vi "Tree.vi"() -> ()   [LabVIEW 2019, in "xy_utilities.lvlib"]
uses:
  xy_utilities.lvlib
  <vilib>/Analysis/NI_AALPro.lvlib
  <vilib>/Analysis/NI_AALBase.lvlib
  <vilib>/measure/NI_MAPro.lvlib
  subVIs/Waveform to XY (single).vi
  subVIs/Waveform to XY (multiple).vi
  subVIs/Interpolate (multiple).vi
  <vilib>/Analysis/6fits.llb/Remove Outliers (Range).vi
  <vilib>/ptbypt/NI_PtbyPt.lvlib
  subVIs/Shift Zero (single).vi
  subVIs/Decimate (single).vi
  subVIs/Subtract float (single).vi
  subVIs/Divide XY (single).vi
  subVIs/Remove Outliers (multiple).vi
  subVIs/Symmetrize (single).vi
  <vilib>/Waveform/WDTOps.llb/WDT Append Waveforms DBL.vi
  <vilib>/Analysis/3filter.llb/Zero Phase Filter (DBL).vi
  <vilib>/Analysis/baseanly.llb/Mean (DBL).vi
  subVIs/Append (double scaler).vi
  subVIs/Interpolate (single).vi
  subVIs/FFT (multiple).vi
  subVIs/Shift Zero (multiple).vi
  subVIs/Add XY (single).vi
  subVIs/Add XY (multiple).vi
  subVIs/XY to Waveform (single).vi
  subVIs/Interpolate Y (multiple).vi
  subVIs/Multiply XY (single).vi
  subVIs/Multiply float (multiple).vi
  subVIs/Square (multiple).vi
  subVIs/Subtract float (multiple).vi
  subVIs/Subset (single).vi
  subVIs/Reverse (multiple).vi
  subVIs/Zero Phase Lowpass Filter (single).vi
  subVIs/Decimate (multiple).vi
  subVIs/Divide float (multiple).vi
  subVIs/Symmetrize (multiple).vi
  subVIs/Restrict X Range (multiple).vi
  subVIs/Resample (single).vi
  subVIs/PS (single).vi
  subVIs/Subtract XY (single).vi
  subVIs/Multiply float (single).vi
  <vilib>/measure/maspectr.llb/FFT Spectrum (Mag-Phase) for 1 Chan.vi
  subVIs/Multiply XY (multiple).vi
  subVIs/Append (double array).vi
  subVIs/Divide XY (multiple).vi
  <vilib>/measure/maspectr.llb/FFT Power Spectrum and PSD for 1 Chan.vi
  subVIs/Get X and Y (single).vi
  subVIs/Remove Outliers (single).vi
  subVIs/FFT (single).vi
  subVIs/Sort (single).vi
  subVIs/Append (multiple).vi
  subVIs/Reverse (single).vi
  subVIs/Divide float (single).vi
  subVIs/Add float (multiple).vi
  subVIs/Savitsky Golay Filter (single).vi
  <vilib>/Analysis/2dsp.llb/Decimate (single shot, DBL).vi
  subVIs/Subset (multiple).vi
  subVIs/XY to Waveform (multiple).vi
  subVIs/Interpolate Y (single).vi
  subVIs/Restrict X Range (single).vi
  subVIs/Derivative (single).vi
  subVIs/Subtract XY (multiple).vi
  subVIs/Square (single).vi
  subVIs/PS (multiple).vi
  subVIs/Swap X and Y (single).vi
  subVIs/Sort (multiple).vi
  <vilib>/measure/maresamp.llb/Resample Waveform (single shot).vi
  subVIs/Resample (multiple).vi
  subVIs/Add float (single).vi
  subVIs/Append (single).vi
  subVIs/Derivative (multiple).vi
  subVIs/Moving Average (single).vi
  <vilib>/Analysis/3filter.llb/Savitzky-Golay Filter (DBL).vi
  subVIs/Swap X and Y (multiple).vi
  subVIs/Get X and Y (multiple).vi
  subVIs/Zero Phase Lowpass Filter (multiple).vi
  subVIs/Moving Average (multiple).vi
  subVIs/Savitsky Golay Filter (multiple).vi
  subVIs/Linear Fit (multiple).vi
  subVIs/Difference Quotient (multiple).vi
  subVIs/Difference Quotient (single).vi
  subVIs/Linear Fit (single).vi
panel:
  out "Array of XY-data":cluster{"X-array":dbl[], "Y-array":dbl[]}[](array[cluster])
  out "XY-data":cluster{"X-array":dbl[], "Y-array":dbl[]}
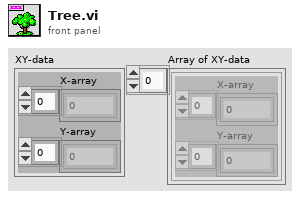
[diagram p1: front panel]
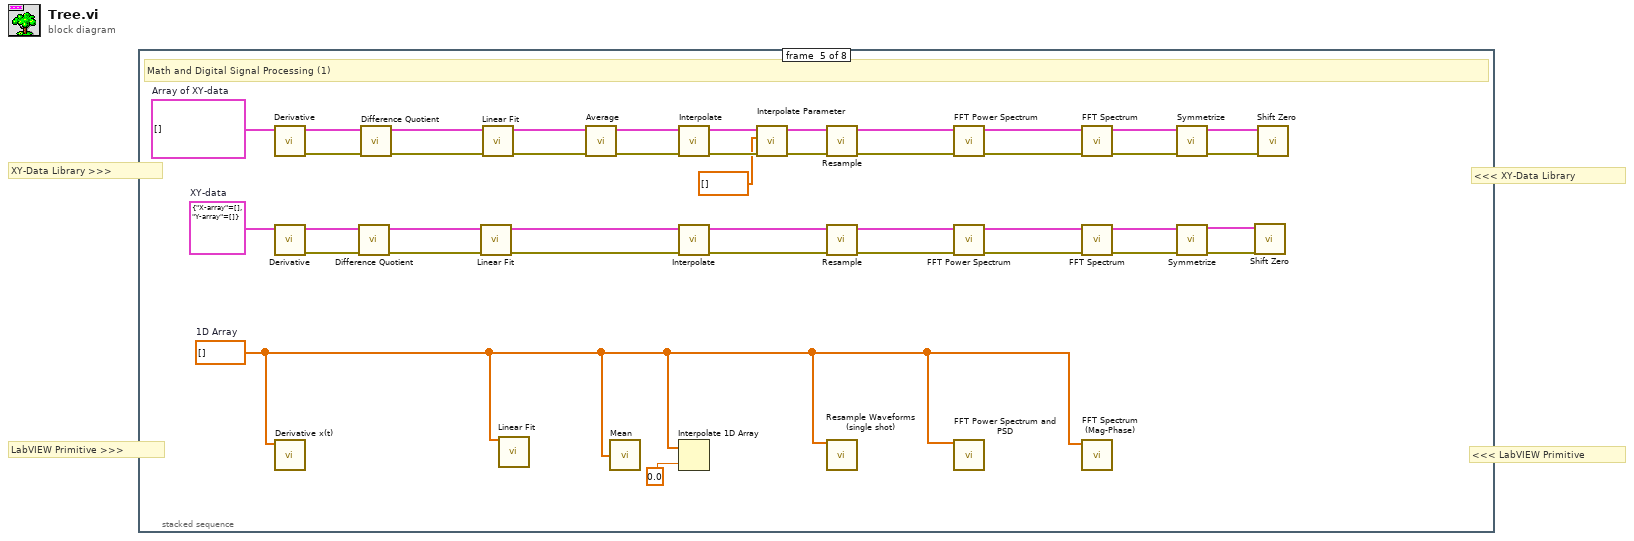
[diagram p0: block diagram]
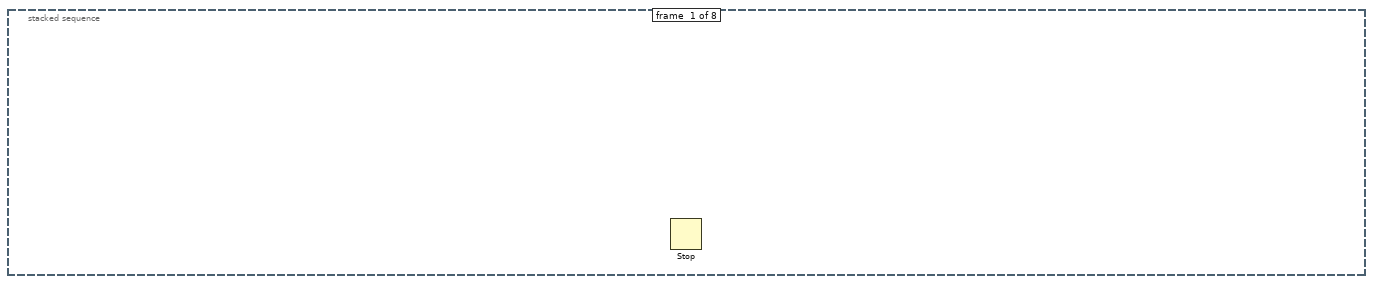
[diagram p2: hidden frame]
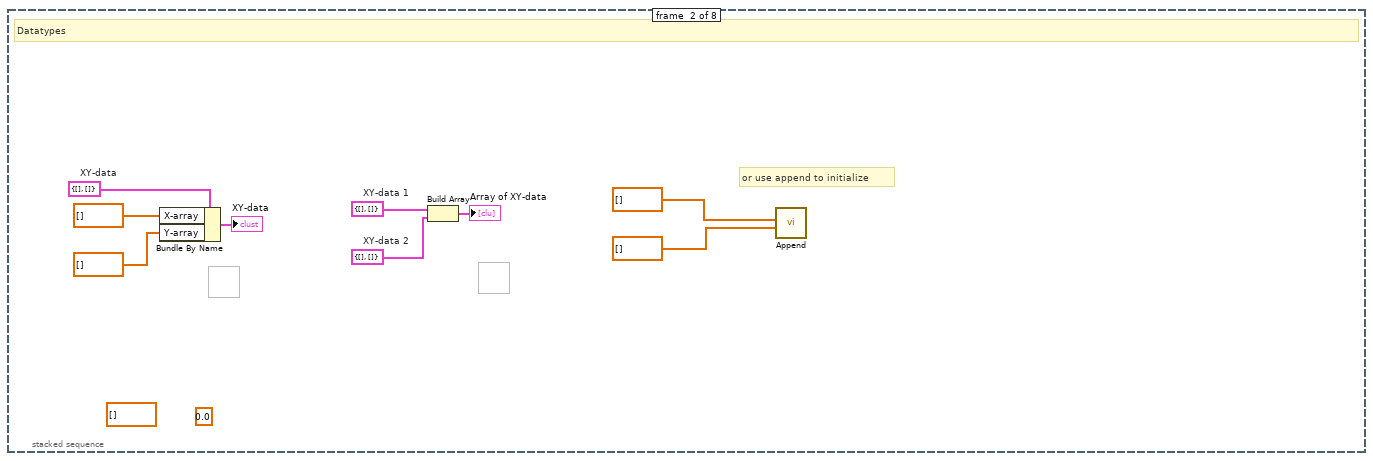
[diagram p3: hidden frame]
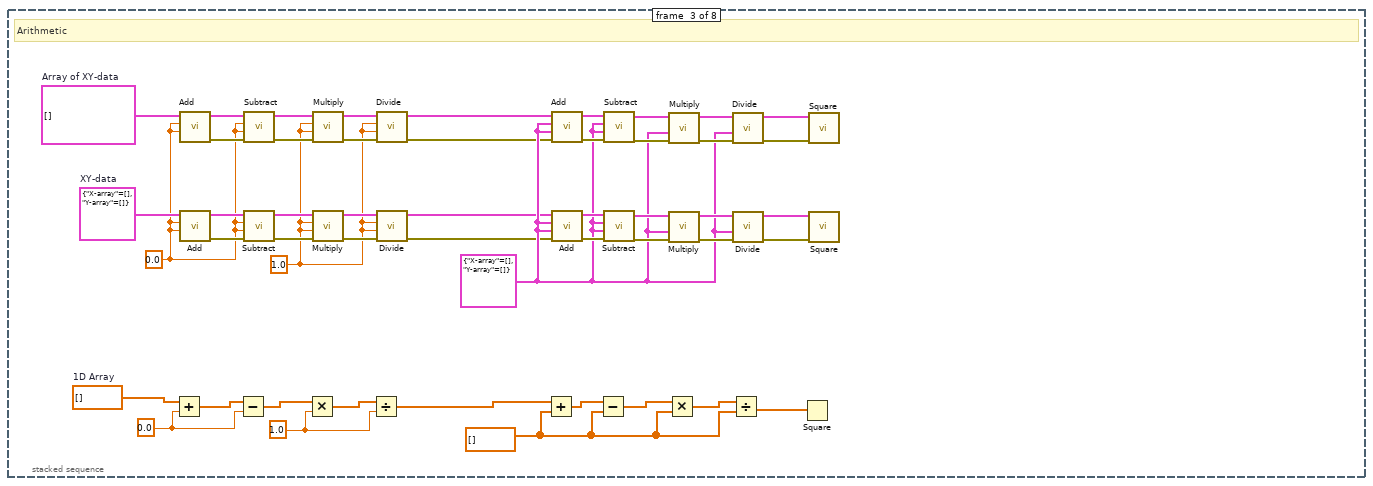
[diagram p4: hidden frame]
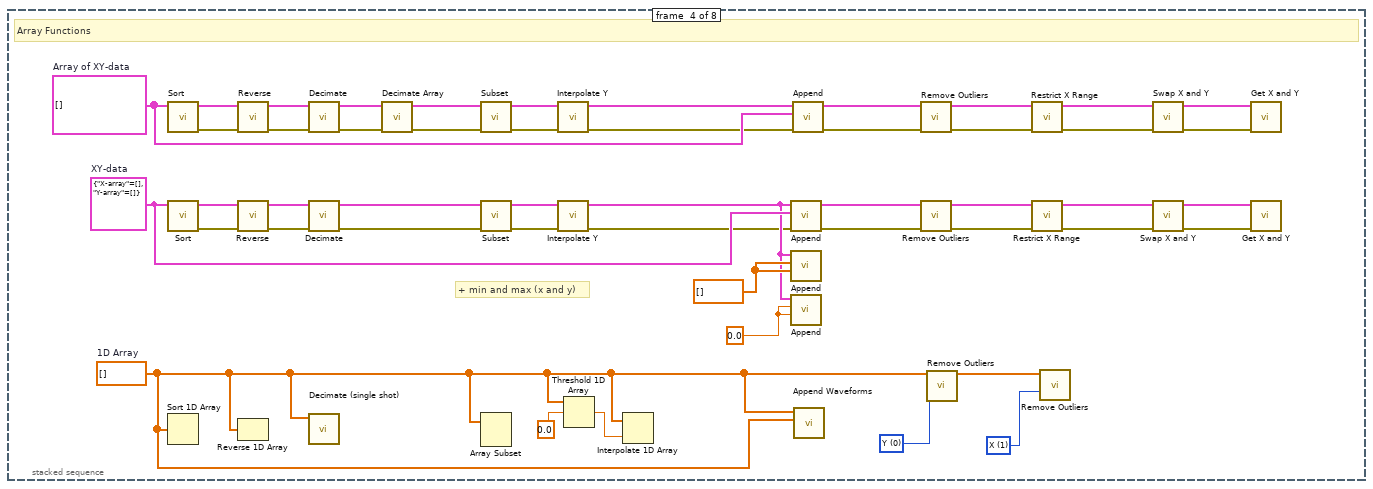
[diagram p5: hidden frame]
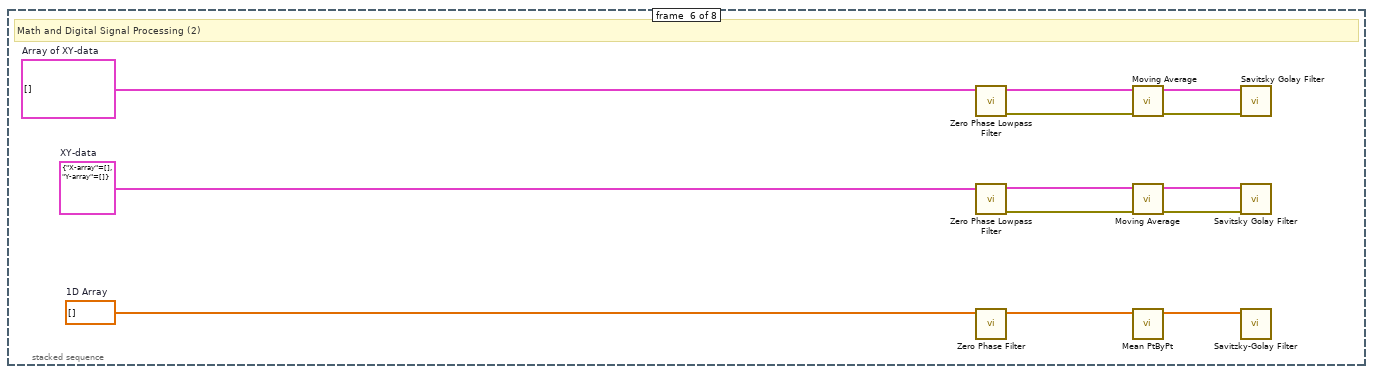
[diagram p6: hidden frame]
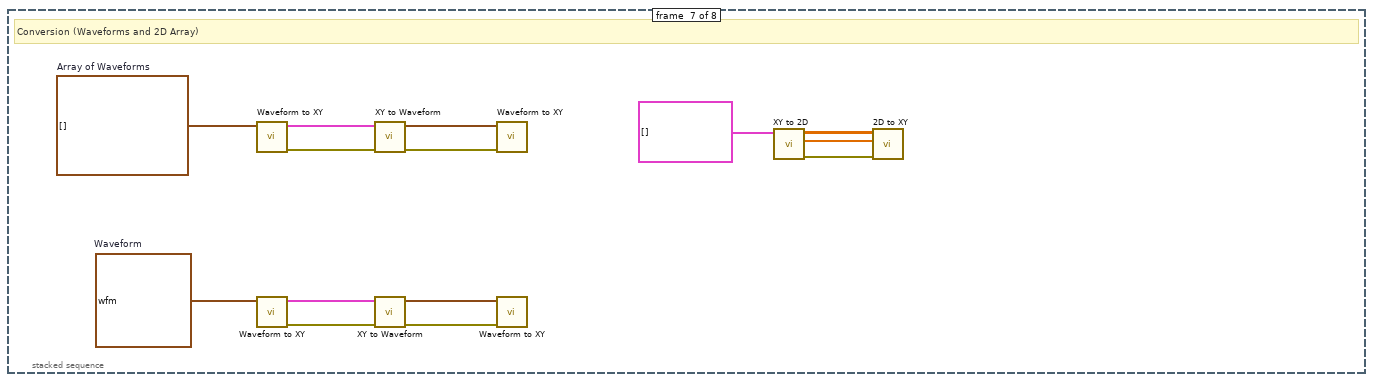
[diagram p7: hidden frame]
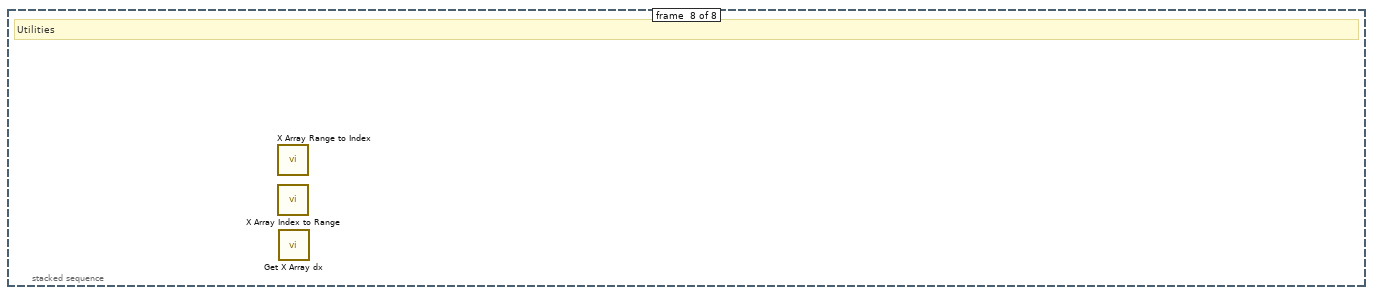
[diagram p8: hidden frame]
diagram:
  # "XY-Data Library >>>"
  # "LabVIEW Primitive >>>"
  # "<<< XY-Data Library"
  # "<<< LabVIEW Primitive"
  n1 = stacked-sequence {
    frame #0 {
      n2 = Stop() -> ()  [unwired: 1 in]
    }
    frame #1 {
      (unwired) 0.0
      (unwired) dbl[] [] ("Y-array")
      w7 = cluster{"X-array":dbl[], "Y-array":dbl[]} {"X-array"=[], "Y-array"=[]}  # XY-data 2
      w8 = cluster{"X-array":dbl[], "Y-array":dbl[]} {"X-array"=[], "Y-array"=[]}  # XY-data 1
      w6 = cluster{"X-array":dbl[], "Y-array":dbl[]} {"X-array"=[], "Y-array"=[]}  # XY-data
      # "or use append to initialize"
      # "Datatypes"
      n3 = Bundle By Name(cluster=w6, "X-array"=dbl[] [], "Y-array"=dbl[] []) -> (→"XY-data":cluster{"X-array":dbl[], "Y-array":dbl[]})
      n4 = Build Array(w8, w7) -> (→"Array of XY-data":cluster{"X-array":dbl[], "Y-array":dbl[]}[])
      n5 = call-poly "Append.vi"("Y-array"=dbl[] [], "X-array"=dbl[] []) -> ()  [unwired: 8 in, 2 out]
    }
    frame #2 {
      w24 = cluster{"X-array":dbl[], "Y-array":dbl[]} {"X-array"=[], "Y-array"=[]} ("XY-data in")
      w33 = 1.0 ("x (0)")
      w42 = 0.0 ("x (0)")
      w21 = dbl[] []
      w35 = 1.0 ("x (0)")
      w36 = 0.0 ("x (0)")
      w10 = dbl[] []  # 1D Array
      w58 = cluster{"X-array":dbl[], "Y-array":dbl[]}[] []  # Array of XY-data
      w57 = cluster{"X-array":dbl[], "Y-array":dbl[]} {"X-array"=[], "Y-array"=[]}  # XY-data
      # "Arithmetic"
      n6 = Add(x=w10, y=w36) -> (x+y=w56:dbl[])
      n7 = call-poly "Add.vi"("y (0)"=w42, "x (0)"=w42, "XY-data"=w58) -> ("error out"=w47:errorcluster, "XY-data out"=w48:cluster{"X-array":dbl[], "Y-array":dbl[]}[])  [unwired: 7 in]
      n8 = call-poly "Add.vi"("y (0)"=w42, "x (0)"=w42, "XY-data"=w57) -> ("error out"=w43:errorcluster, "XY-data out"=w44:cluster{"X-array":dbl[], "Y-array":dbl[]})  [unwired: 7 in]
      n9 = Subtract(x=w56, y=w36) -> (x-y=w55:dbl[])
      n10 = call-poly "Subtract.vi"("error in (no error)"=w47, "y (0)"=w42, "x (0)"=w42, "XY-data"=w48) -> ("error out"=w45:errorcluster, "XY-data out"=w46:cluster{"X-array":dbl[], "Y-array":dbl[]}[])  [unwired: 6 in]
      n11 = call-poly "Subtract.vi"("error in (no error)"=w43, "y (0)"=w42, "x (0)"=w42, "XY-data"=w44) -> ("error out"=w50:errorcluster, "XY-data out"=w51:cluster{"X-array":dbl[], "Y-array":dbl[]})  [unwired: 6 in]
      n12 = Multiply(x=w55, y=w35) -> (x*y=w37:dbl[])
      n13 = call-poly "Multiply.vi"("error in (no error)"=w45, "y (1)"=w33, "x (1)"=w33, "XY-data"=w46) -> ("error out"=w52:errorcluster, "XY-data out"=w54:cluster{"X-array":dbl[], "Y-array":dbl[]}[])  [unwired: 6 in]
      n14 = call-poly "Multiply.vi"("error in (no error)"=w50, "y (1)"=w33, "x (1)"=w33, "XY-data"=w51) -> ("error out"=w49:errorcluster, "XY-data out"=w53:cluster{"X-array":dbl[], "Y-array":dbl[]})  [unwired: 6 in]
      n15 = Divide(x=w37, y=w35) -> (x/y=w16:dbl[])
      n16 = call-poly "Divide.vi"("error in (no error)"=w52, "y (1)"=w33, "x (1)"=w33, "XY-data"=w54) -> ("error out"=w19:errorcluster, "XY-data out"=w20:cluster{"X-array":dbl[], "Y-array":dbl[]}[])  [unwired: 6 in]
      n17 = call-poly "Divide.vi"("error in (no error)"=w49, "y (1)"=w33, "x (1)"=w33, "XY-data"=w53) -> ("error out"=w17:errorcluster, "XY-data out"=w18:cluster{"X-array":dbl[], "Y-array":dbl[]})  [unwired: 6 in]
      n18 = Add(x=w16, y=w21) -> (x+y=w34:dbl[])
      n19 = call-poly "Add.vi"("error in (no error)"=w19, "y"=w24, "x"=w24, "XY-data"=w20) -> ("error out"=w40:errorcluster, "XY-data out"=w39:cluster{"X-array":dbl[], "Y-array":dbl[]}[])  [unwired: 6 in]
      n20 = call-poly "Add.vi"("error in (no error)"=w17, "y"=w24, "x"=w24, "XY-data"=w18) -> ("error out"=w38:errorcluster, "XY-data out"=w41:cluster{"X-array":dbl[], "Y-array":dbl[]})  [unwired: 6 in]
      n21 = Subtract(x=w34, y=w21) -> (x-y=w22:dbl[])
      n22 = call-poly "Subtract.vi"("error in (no error)"=w40, "y"=w24, "x"=w24, "XY-data"=w39) -> ("error out"=w27:errorcluster, "XY-data out"=w28:cluster{"X-array":dbl[], "Y-array":dbl[]}[])  [unwired: 6 in]
      n23 = call-poly "Subtract.vi"("error in (no error)"=w38, "y"=w24, "x"=w24, "XY-data"=w41) -> ("error out"=w25:errorcluster, "XY-data out"=w26:cluster{"X-array":dbl[], "Y-array":dbl[]})  [unwired: 6 in]
      n24 = Multiply(x=w22, y=w21) -> (x*y=w23:dbl[])
      n25 = call-poly "Multiply.vi"("error in (no error)"=w27, "y"=w24, "XY-data"=w28) -> ("error out"=w31:errorcluster, "XY-data out"=w29:cluster{"X-array":dbl[], "Y-array":dbl[]}[])  [unwired: 7 in]
      n26 = call-poly "Multiply.vi"("error in (no error)"=w25, "y"=w24, "XY-data"=w26) -> ("error out"=w32:errorcluster, "XY-data out"=w30:cluster{"X-array":dbl[], "Y-array":dbl[]})  [unwired: 7 in]
      n27 = Divide(x=w23, y=w21) -> (x/y=w11:dbl[])
      n28 = call-poly "Divide.vi"("error in (no error)"=w31, "y"=w24, "XY-data"=w29) -> ("error out"=w14:errorcluster, "XY-data out"=w15:cluster{"X-array":dbl[], "Y-array":dbl[]}[])  [unwired: 7 in]
      n29 = call-poly "Divide.vi"("error in (no error)"=w32, "y"=w24, "XY-data"=w30) -> ("error out"=w12:errorcluster, "XY-data out"=w13:cluster{"X-array":dbl[], "Y-array":dbl[]})  [unwired: 7 in]
      n30 = Square(x=w11) -> ()  [unwired: 1 out]
      n31 = call-poly "Square.vi"("error in (no error)"=w14, "XY-data"=w15) -> ()  [unwired: 8 in, 2 out]
      n32 = call-poly "Square.vi"("error in (no error)"=w12, "XY-data"=w13) -> ()  [unwired: 8 in, 2 out]
    }
    frame #3 {
      w76 = dbl[] [] ("1D Array")
      w77 = u16 1 items=["Y", "X", "X and Y"] ("range type")
      w78 = u16 0 items=["Y", "X", "X and Y"] ("range type")
      w75 = 0.0 ("threshold y")
      w71 = dbl[] []  # 1D Array
      w73 = cluster{"X-array":dbl[], "Y-array":dbl[]}[] []  # Array of XY-data
      w74 = cluster{"X-array":dbl[], "Y-array":dbl[]} {"X-array"=[], "Y-array"=[]}  # XY-data
      # "+ min and max (x and y)"
      # "Array Functions"
      n33 = call-poly "Sort.vi"("XY-data"=w73) -> ("error out"=w101:errorcluster, "Sorted XY-data out"=w102:cluster{"X-array":dbl[], "Y-array":dbl[]}[])  [unwired: 9 in]
      n34 = call-poly "Sort.vi"("XY-data"=w74) -> ("error out"=w97:errorcluster, "Sorted XY-data out"=w98:cluster{"X-array":dbl[], "Y-array":dbl[]})  [unwired: 9 in]
      n35 = Sort 1D Array(array=w71) -> ()  [unwired: 1 out]
      n36 = call-poly "Reverse.vi"("error in (no error)"=w101, "XY-data"=w102) -> ("error out"=w99:errorcluster, "Reversed XY-data out"=w100:cluster{"X-array":dbl[], "Y-array":dbl[]}[])  [unwired: 8 in]
      n37 = call-poly "Reverse.vi"("error in (no error)"=w97, "XY-data"=w98) -> ("error out"=w104:errorcluster, "Reversed XY-data out"=w103:cluster{"X-array":dbl[], "Y-array":dbl[]})  [unwired: 8 in]
      n38 = Reverse 1D Array(array=w71) -> ()  [unwired: 1 out]
      n39 = call-poly "Decimate.vi"("error in (no error)"=w99, "XY-data"=w100) -> ("error out"=w96:errorcluster, "Decimated XY-data out"=w95:cluster{"X-array":dbl[], "Y-array":dbl[]}[])  [unwired: 8 in]
      n40 = call-poly "Decimate.vi"("error in (no error)"=w104, "XY-data"=w103) -> ("error out"=w105:errorcluster, "Decimated XY-data out"=w106:cluster{"X-array":dbl[], "Y-array":dbl[]})  [unwired: 8 in]
      n41 = call-poly <vilib>:"Decimate (single shot).vi"("X"=w71) -> ()  [unwired: 9 in, 2 out]
      n42 = call "Decimate Array.vi"("error in (no error)"=w96, "XY-data"=w95) -> ("error out"=w94:errorcluster, "Decimated XY-data out"=w93:cluster{"X-array":dbl[], "Y-array":dbl[]}[])  [unwired: 8 in]
      n43 = call-poly "Subset.vi"("error in (no error)"=w94, "XY-data"=w93) -> ("error out"=w91:errorcluster, "Subset XY-data out"=w92:cluster{"X-array":dbl[], "Y-array":dbl[]}[])  [unwired: 8 in]
      n44 = call-poly "Subset.vi"("error in (no error)"=w105, "XY-data"=w106) -> ("error out"=w89:errorcluster, "XY-data out"=w90:cluster{"X-array":dbl[], "Y-array":dbl[]})  [unwired: 8 in]
      n45 = Array Subset "Array Subset"(array=w71) -> ()  [unwired: 2 in, 1 out]
      n46 = call-poly "Interpolate Y.vi"("error in (no error)"=w91, "XY-data"=w92) -> ("error out"=w69:errorcluster, "XY-data out"=w70:cluster{"X-array":dbl[], "Y-array":dbl[]}[])  [unwired: 7 in, 1 out]
      n47 = call-poly "Interpolate Y.vi"("error in (no error)"=w89, "XY-data"=w90) -> ("error out"=w67:errorcluster, "XY-data out"=w68:cluster{"X-array":dbl[], "Y-array":dbl[]})  [unwired: 7 in, 1 out]
      n48 = Threshold 1D Array(2:0.0 ("threshold y"), 3:w71) -> (0:w88:dbl)  [unwired: 1 in]
      n49 = Interpolate 1D Array(1:w88, 2:w71) -> ()  [unwired: 1 out]
      n50 = call-poly "Append.vi"("error in (no error)"=w67, "XY-data (B)"=w74, "XY-data (A)"=w68) -> ("error out"=w82:errorcluster, "XY-data out"=w83:cluster{"X-array":dbl[], "Y-array":dbl[]})  [unwired: 7 in]
      n51 = call-poly "Append.vi"("Y-array"=w76, "X-array"=w76, "XY-data (A)"=w68) -> ()  [unwired: 7 in, 2 out]
      n52 = call-poly "Append.vi"("Y"=w75, "X"=w75, "XY-data (A)"=w68) -> ()  [unwired: 7 in, 2 out]
      n53 = call-poly "Append.vi"("error in (no error)"=w69, "XY-data (B)"=w73, "XY-data (A)"=w70) -> ("error out"=w80:errorcluster, "XY-data out"=w87:cluster{"X-array":dbl[], "Y-array":dbl[]}[])  [unwired: 7 in]
      n54 = call-poly <vilib>:"Append Waveforms.vi"("waveform B"=w71, "waveform A"=w71) -> ()  [unwired: 8 in, 2 out]
      n55 = call-poly <vilib>:"Remove Outliers.vi"("error in (no error)"=w80, "XY-data"=w87) -> ("error out"=w85:errorcluster, "XY-data out"=w86:cluster{"X-array":dbl[], "Y-array":dbl[]}[])  [unwired: 8 in]
      n56 = call-poly <vilib>:"Remove Outliers.vi"("error in (no error)"=w82, "XY-data"=w83) -> ("error out"=w84:errorcluster, "XY-data out"=w81:cluster{"X-array":dbl[], "Y-array":dbl[]})  [unwired: 8 in]
      n57 = call-poly <vilib>:"Remove Outliers.vi"("Y"=w71, "range type"=w78) -> ("Y Out"=w79:dbl[])  [unwired: 9 in, 4 out]
      n58 = call-poly "Restrict X Range.vi"("error in (no error)"=w85, "XY-data"=w86) -> ("error out"=w63:errorcluster, "XY-data out"=w66:cluster{"X-array":dbl[], "Y-array":dbl[]}[])  [unwired: 8 in]
      n59 = call-poly "Restrict X Range.vi"("error in (no error)"=w84, "XY-data"=w81) -> ("error out"=w59:errorcluster, "XY-data out"=w62:cluster{"X-array":dbl[], "Y-array":dbl[]})  [unwired: 8 in]
      n60 = call-poly <vilib>:"Remove Outliers.vi"("Y"=w79, "range type"=w77) -> ()  [unwired: 9 in, 5 out]
      n61 = call-poly "Swap X and Y.vi"("error in (no error)"=w63, "XY-data"=w66) -> ("error out"=w64:errorcluster, "XY-data out"=w65:cluster{"X-array":dbl[], "Y-array":dbl[]}[])  [unwired: 8 in]
      n62 = call-poly "Swap X and Y.vi"("error in (no error)"=w59, "XY-data"=w62) -> ("error out"=w60:errorcluster, "XY-data out"=w61:cluster{"X-array":dbl[], "Y-array":dbl[]})  [unwired: 8 in]
      n63 = call-poly "Get X and Y.vi"("error in (no error)"=w64, "XY-data"=w65) -> ()  [unwired: 6 in, 4 out]
      n64 = call-poly "Get X and Y.vi"("error in (no error)"=w60, "XY-data"=w61) -> ()  [unwired: 6 in, 4 out]
    }
    frame #4 {
      w107 = dbl[] []  # 1D Array
      w136 = cluster{"X-array":dbl[], "Y-array":dbl[]}[] []  # Array of XY-data
      w135 = cluster{"X-array":dbl[], "Y-array":dbl[]} {"X-array"=[], "Y-array"=[]}  # XY-data
      # "Math and Digital Signal Processing (1)"
      n65 = call-poly "Derivative.vi"("XY-data"=w136) -> ("error out"=w118:errorcluster, "XY-data out"=w119:cluster{"X-array":dbl[], "Y-array":dbl[]}[])  [unwired: 8 in, 1 out]
      n66 = call-poly "Derivative.vi"("XY-data"=w135) -> ("error out"=w108:errorcluster, "XY-data out"=w112:cluster{"X-array":dbl[], "Y-array":dbl[]})  [unwired: 8 in, 1 out]
      n67 = call <vilib>:"Derivative x(t).vi"("X"=w107) -> ()  [unwired: 9 in, 2 out]
      n68 = call-poly "Difference Quotient.vi"("error in (no error)"=w108, "XY-data"=w112) -> ("error out"=w113:errorcluster, "XY-data out"=w111:cluster{"X-array":dbl[], "Y-array":dbl[]})  [unwired: 7 in, 1 out]
      n69 = call-poly "Difference Quotient.vi"("error in (no error)"=w118, "XY-data"=w119) -> ("error out"=w116:errorcluster, "XY-data out"=w117:cluster{"X-array":dbl[], "Y-array":dbl[]}[])  [unwired: 7 in, 1 out]
      n70 = call-poly <vilib>:"Linear Fit.vi"("error in (no error)"=w113, "XY-data"=w111) -> ("error out"=w109:errorcluster, "XY-data out"=w110:cluster{"X-array":dbl[], "Y-array":dbl[]})  [unwired: 3 in, 5 out]
      n71 = call-poly <vilib>:"Linear Fit.vi"("error in (no error)"=w116, "XY-data"=w117) -> ("error out"=w115:errorcluster, "XY-data out"=w114:cluster{"X-array":dbl[], "Y-array":dbl[]}[])  [unwired: 3 in, 5 out]
      n72 = call <vilib>:"Linear Fit.vi"("Y"=w107) -> ()  [unwired: 10 in, 5 out]
      n73 = call "Average.vi"("error in (no error)"=w115, "XY-data"=w114) -> ("error out"=w141:errorcluster, "XY-data out"=w142:cluster{"X-array":dbl[], "Y-array":dbl[]}[])  [unwired: 7 in, 1 out]
      n74 = call-poly <vilib>:"Mean.vi"("X"=w107) -> ()  [unwired: 2 out]
      n75 = call-poly "Interpolate.vi"("error in (no error)"=w141, "XY-data"=w142) -> ("error out"=w123:errorcluster, "Interpolated XY-data out"=w125:cluster{"X-array":dbl[], "Y-array":dbl[]}[])  [unwired: 8 in]
      n76 = call-poly "Interpolate.vi"("error in (no error)"=w109, "XY-data"=w110) -> ("error out"=w143:errorcluster, "Interpolated XY-data out"=w126:cluster{"X-array":dbl[], "Y-array":dbl[]})  [unwired: 8 in]
      n77 = Interpolate 1D Array(1:0.0 ("fractional index or x"), 2:w107) -> ()  [unwired: 1 out]
      n78 = call "Interpolate Parameter.vi"("error in (no error)"=w123, "Parameter-array"=dbl[] [] ("1D Array"), "XY-data"=w125) -> ("error out"=w122:errorcluster, "Interpolated XY-data out"=w124:cluster{"X-array":dbl[], "Y-array":dbl[]}[])  [unwired: 6 in, 1 out]
      n79 = call-poly "Resample.vi"("error in (no error)"=w122, "XY-data"=w124) -> ("error out"=w139:errorcluster, "Resampled XY-data out"=w140:cluster{"X-array":dbl[], "Y-array":dbl[]}[])  [unwired: 8 in]
      n80 = call-poly "Resample.vi"("error in (no error)"=w143, "XY-data"=w126) -> ("error out"=w137:errorcluster, "Resampled XY-data out"=w138:cluster{"X-array":dbl[], "Y-array":dbl[]})  [unwired: 8 in]
      n81 = call-poly <vilib>:"Resample Waveforms (single shot).vi"("waveform in"=w107) -> ()  [unwired: 11 in, 4 out]
      n82 = call-poly "FFT Power Spectrum.vi"("error in (no error)"=w139, "XY-data"=w140) -> ("error out"=w145:errorcluster, "XY-data out"=w146:cluster{"X-array":dbl[], "Y-array":dbl[]}[])  [unwired: 7 in, 1 out]
      n83 = call-poly "FFT Power Spectrum.vi"("error in (no error)"=w137, "XY-data"=w138) -> ("error out"=w144:errorcluster, "XY-data out"=w147:cluster{"X-array":dbl[], "Y-array":dbl[]})  [unwired: 7 in, 1 out]
      n84 = call-poly <vilib>:"FFT Power Spectrum and PSD.vi"("time signal"=w107) -> ()  [unwired: 7 in, 4 out]
      n85 = call-poly "FFT Spectrum.vi"("error in (no error)"=w145, "XY-data"=w146) -> ("error out"=w131:errorcluster, "XY-data out"=w134:cluster{"X-array":dbl[], "Y-array":dbl[]}[])  [unwired: 6 in, 2 out]
      n86 = call-poly "FFT Spectrum.vi"("error in (no error)"=w144, "XY-data"=w147) -> ("error out"=w132:errorcluster, "XY-data out"=w133:cluster{"X-array":dbl[], "Y-array":dbl[]})  [unwired: 6 in, 2 out]
      n87 = call-poly <vilib>:"FFT Spectrum (Mag-Phase).vi"("time signal"=w107) -> ()  [unwired: 6 in, 5 out]
      n88 = call-poly "Symmetrize.vi"("error in (no error)"=w131, "XY-data"=w134) -> ("error out"=w128:errorcluster, "XY-data out"=w127:cluster{"X-array":dbl[], "Y-array":dbl[]}[])  [unwired: 6 in, 2 out]
      n89 = call-poly "Symmetrize.vi"("error in (no error)"=w132, "XY-data"=w133) -> ("error out"=w130:errorcluster, "XY-data out"=w129:cluster{"X-array":dbl[], "Y-array":dbl[]})  [unwired: 6 in, 2 out]
      n90 = call-poly "Shift Zero.vi"("error in (no error)"=w130, "XY-data"=w129) -> ()  [unwired: 8 in, 2 out]
      n91 = call-poly "Shift Zero.vi"("error in (no error)"=w128, "XY-data"=w127) -> ()  [unwired: 8 in, 2 out]
    }
    frame #5 {
      w149 = dbl[] []  # 1D Array
      w158 = cluster{"X-array":dbl[], "Y-array":dbl[]}[] []  # Array of XY-data
      w159 = cluster{"X-array":dbl[], "Y-array":dbl[]} {"X-array"=[], "Y-array"=[]}  # XY-data
      # "Math and Digital Signal Processing (2)"
      n92 = call-poly "Zero Phase Lowpass Filter.vi"("XY-data"=w158) -> ("error out"=w156:errorcluster, "XY-data out"=w157:cluster{"X-array":dbl[], "Y-array":dbl[]}[])  [unwired: 9 in]
      n93 = call-poly "Zero Phase Lowpass Filter.vi"("XY-data"=w159) -> ("error out"=w155:errorcluster, "XY-data out"=w154:cluster{"X-array":dbl[], "Y-array":dbl[]})  [unwired: 9 in]
      n94 = call-poly <vilib>:"Zero Phase Filter.vi"("X"=w149) -> ("Filtered X"=w148:dbl[])  [unwired: 9 in, 1 out]
      n95 = call-poly "Moving Average.vi"("error in (no error)"=w156, "XY-data"=w157) -> ("error out"=w152:errorcluster, "XY-data out"=w153:cluster{"X-array":dbl[], "Y-array":dbl[]}[])  [unwired: 8 in]
      n96 = call-poly "Moving Average.vi"("error in (no error)"=w155, "XY-data"=w154) -> ("error out"=w151:errorcluster, "XY-data out"=w150:cluster{"X-array":dbl[], "Y-array":dbl[]})  [unwired: 8 in]
      n97 = call <vilib>:"Mean PtByPt.vi"() -> ()  [unwired: 4 in, 2 out]
      n98 = call-poly "Savitsky Golay Filter.vi"("error in (no error)"=w152, "XY-data"=w153) -> ()  [unwired: 8 in, 2 out]
      n99 = call-poly "Savitsky Golay Filter.vi"("error in (no error)"=w151, "XY-data"=w150) -> ()  [unwired: 8 in, 2 out]
      n100 = call-poly <vilib>:"Savitzky-Golay Filter.vi"("X"=w148) -> ()  [unwired: 9 in, 2 out]
    }
    frame #6 {
      w172 = waveform(dbl)[] []  # Array of Waveforms
      w173 = waveform(dbl) {"t0"=timestamp(0 s since 1904-01-01), "dt"=1.0, "Y"=[]}  # Waveform
      # "Conversion (Waveforms and 2D Array)"
      n101 = call-poly "Waveform to XY.vi"("Waveform in"=w172) -> ("error out"=w170:errorcluster, "XY-data out"=w164:cluster{"X-array":dbl[], "Y-array":dbl[]}[])  [unwired: 9 in]
      n102 = call-poly "Waveform to XY.vi"("Waveform in"=w173) -> ("error out"=w166:errorcluster, "XY-data out"=w171:cluster{"X-array":dbl[], "Y-array":dbl[]})  [unwired: 9 in]
      n103 = call-poly "XY to Waveform.vi"("error in (no error)"=w170, "XY-data in"=w164) -> ("error out"=w167:errorcluster, "Waveform out"=w169:waveform(dbl)[])  [unwired: 7 in, 1 out]
      n104 = call-poly "XY to Waveform.vi"("error in (no error)"=w166, "XY-data in"=w171) -> ("error out"=w165:errorcluster, "Waveform out"=w168:waveform(dbl))  [unwired: 7 in, 1 out]
      n105 = call-poly "Waveform to XY.vi"("error in (no error)"=w167, "Waveform in"=w169) -> ()  [unwired: 8 in, 2 out]
      n106 = call-poly "Waveform to XY.vi"("error in (no error)"=w165, "Waveform in"=w168) -> ()  [unwired: 8 in, 2 out]
      n107 = call "XY to 2D.vi"("XY-data"=cluster{"X-array":dbl[], "Y-array":dbl[]}[] []) -> ("error out"=w160:errorcluster, "X Array"=w161:dbl[], "2D Y Array"=w162:dbl[][])  [unwired: 7 in, 1 out]
      n108 = call "2D to XY.vi"("error in (no error)"=w160, "X Array"=w161, "2D Y Array"=w162) -> ()  [unwired: 7 in, 2 out]
    }
    frame #7 {
      # "Utilities"
      n109 = call "X Array Range to Index.vi"() -> ()  [unwired: 3 in, 1 out]
      n110 = call "X Array Index to Range.vi"() -> ()  [unwired: 3 in, 1 out]
      n111 = call "Get X Array dx.vi"() -> ()  [unwired: 8 in, 4 out]
    }
  }
